vi "Alicat Comm Example.vi"() -> ()   [LabVIEW 2014, in "Alicat.lvlib"]
uses:
  Alicat.lvlib
  AlicatCommBank.lvclass
  MC/Alicat_MC.lvclass
  Alicat.lvclass
  Controls/Gas.ctl
  Controls/CtlSetup.ctl
  Data/MC/AlicatMCData.lvclass
panel:
  in  "SP1":dbl
  out "T 2":sgl
  out "P 2":sgl
  in  "SP":dbl[](array[numeric])
  out "P":sgl[](array[numeric])
  out "T":sgl[](array[numeric])
  in  "stop":bool
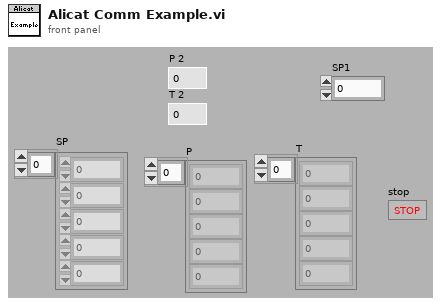
[diagram p1: front panel]
types:
  T1 = typedef "Alicat.lvlib/Alicat.lvclass/CtlSetup.ctl" = cluster{"Name":string, "Address":string, "fullScale":dbl, "Gas":T2}
  T2 = typedef "Alicat.lvlib/Alicat.lvclass/Gas.ctl" = enum16{"Air", "Ar", "CH4", "CO", "CO2", "C2H6", "H2", "He", "N2", "NO", "Ne", "O2", "C3H8", "n-C4H10", "C2H2", "C2H4", "i-C2H10", "Kr", "Xe"}
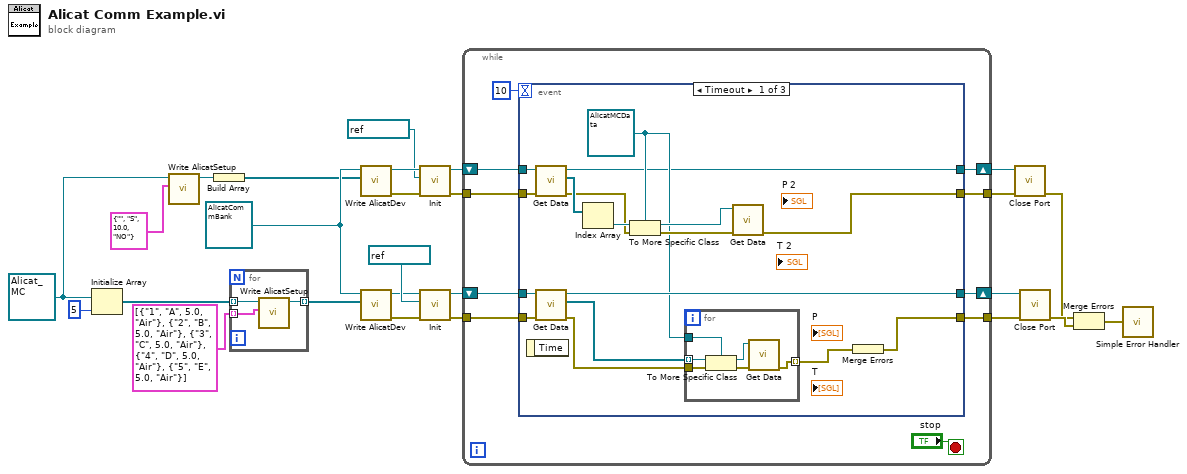
[diagram p0: block diagram]
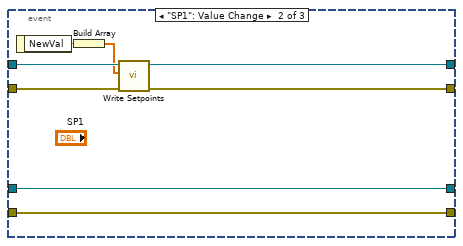
[diagram p2: hidden frame]
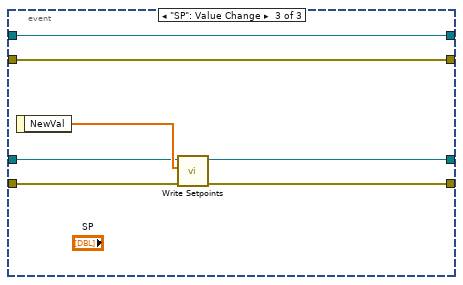
[diagram p3: hidden frame]
diagram:
  w15 = refnum<class "Alicat_MC.lvclass"> refnum ("Alicat_MC.lvclass")
  w12 = refnum<class "AlicatCommBank.lvclass"> refnum ("AlicatCommBank in")
  n1 = Initialize Array(w15, 5 ("dimension size")) -> (w18:refnum<class "Alicat_MC.lvclass">[])
  n2 = call "Write AlicatSetup.vi"("AlicatSetup"=T1 {"Name"="", "Address"="S", "fullScale"=10.0, "Gas"=enum."NO"}, "Alicat in"=w15) -> ("Alicat out"=w13:refnum<class "Alicat_MC.lvclass">)  [unwired: 8 in, 1 out]
  n3 = Build Array(w13) -> (w11:refnum<class "Alicat_MC.lvclass">[])
  n4 = for {
    tunnel: w18 -> [w29] mode=indexing
    tunnel: [w28] -> w17 mode=indexing
    tunnel: T1[] [{"Name"="1", "Address"="A", "fullScale"=5.0, "Gas"=enum."Air"}, {"Name"="2", "Address"="B", "fullScale"=5.0, "Gas"=enum."Air"}, {"Name"="3", "Address"="C", "fullScale"=5.0, "Gas"=enum."Air"}, {"Name"="4", "Address"="D", "fullScale"=5.0, "Gas"=enum."Air"}, {"Name"="5", "Address"="E", "fullScale"=5.0, "Gas"=enum."Air"}] -> [w27] mode=indexing
    n5 = call "Write AlicatSetup.vi"("AlicatSetup"=w27, "Alicat in"=w29) -> ("Alicat out"=w28:refnum<class "Alicat_MC.lvclass">)  [unwired: 8 in, 1 out]
  }
  n6 = call "Write AlicatDev.vi"("AlicatDev"=w11, "AlicatCommBank in"=w12) -> ("error out"=w7:errorcluster, "AlicatCommBank out"=w8:refnum<class "AlicatCommBank.lvclass">)  [unwired: 8 in]
  n7 = call "Write AlicatDev.vi"("AlicatDev"=w17, "AlicatCommBank in"=w12) -> ("error out"=w23:errorcluster, "AlicatCommBank out"=w25:refnum<class "AlicatCommBank.lvclass">)  [unwired: 8 in]
  n8 = call-dynamic "Init.vi"("error in"=w7, "Port"=refnum<visa-resource-name> "COM5", "AlicatCommBank in"=w8) -> ("error out"=w4:errorcluster, "AlicatCommBank out"=w5:refnum<class "AlicatCommBank.lvclass">)  [unwired: 7 in]
  n9 = call-dynamic "Init.vi"("error in"=w23, "Port"=refnum<visa-resource-name> "COM3", "AlicatCommBank in"=w25) -> ("error out"=w21:errorcluster, "AlicatCommBank out"=w22:refnum<class "AlicatCommBank.lvclass">)  [unwired: 7 in]
  n10 = while {
    tunnel: w21 -> [w38]
    tunnel: [w35] -> w19
    tunnel: w4 -> [w32]
    tunnel: [w30] -> w9
    shift-right: [w36] -> w20
    shift-left: w22 -> [w39]
    shift-right: [w31] -> w10
    shift-left: w5 -> [w33]
    stop <- "stop" stop-if-true
    n11 = event shown="[0] Timeout" {
      selector: _ -> [_ _ _]
      dyn-events: _ -> [_ _ _]
      timeout: 10 -> [_ _ _]
      tunnel: w39 -> [w56 w70 w76]
      tunnel: w38 -> [w55 w69 w75]
      tunnel: [w54 w70 w73] -> w36
      tunnel: [w40 w69 w74] -> w35
      tunnel: w33 -> [w52 w68 w72]
      tunnel: w32 -> [w51 w67 w71]
      tunnel: [w45 w65 w72] -> w31
      tunnel: [w43 w66 w71] -> w30
      event Timeout {
        w46 = refnum<class "AlicatMCData.lvclass"> refnum ("Alicat.lvlib:AlicatMCData.lvclass")
        n12 = event-data() -> ()  [unwired: 1 in, 1 out]
        n13 = call-dynamic "Get Data.vi"("error in"=w51, "AlicatCommBank in"=w52) -> ("error out"=w44:errorcluster, "DataOut"=w48:refnum<class "Data.lvclass">[], "AlicatCommBank out"=w45:refnum<class "AlicatCommBank.lvclass">)  [unwired: 7 in]
        n14 = call-dynamic "Get Data.vi"("error in"=w55, "AlicatCommBank in"=w56) -> ("error out"=w42:errorcluster, "DataOut"=w53:refnum<class "Data.lvclass">[], "AlicatCommBank out"=w54:refnum<class "AlicatCommBank.lvclass">)  [unwired: 7 in]
        n15 = Index Array(array=w48) -> (element=w47:refnum<class "Data.lvclass">)  [unwired: 1 in]
        n16 = To More Specific Class(target class=w46, reference=w47, error in=w44) -> (specific class reference=w50:refnum<class "AlicatMCData.lvclass">, error out=w49:errorcluster)
        n17 = for {
          tunnel: w53 -> [w61] mode=indexing
          tunnel: w46 -> [w60]
          tunnel: w42 -> [w58]
          tunnel: [w57] -> w41 mode=indexing
          n18 = To More Specific Class(target class=w60, reference=w61, error in=w58) -> (specific class reference=w59:refnum<class "AlicatMCData.lvclass">, error out=w62:errorcluster)
          n19 = call "Get Data.vi"("error in"=w62, "AlicatMData in"=w59) -> ("error out"=w57:errorcluster)  [unwired: 7 in, 2 out]
        }
        n20 = call "Get Data.vi"("error in"=w49, "AlicatMData in"=w50) -> ("error out"=w43:errorcluster)  [unwired: 7 in, 2 out]
        n21 = Merge Errors(w41) -> (w40:errorcluster)
      }
      event "SP1": Value Change {
        n22 = event-data() -> ("NewVal"=w64:dbl)  [unwired: 1 in]
        n23 = Build Array(w64) -> (w63:dbl[])
        n24 = call-dynamic "Write Setpoints.vi"("error in"=w67, "Setpoints"=w63, "AlicatCommBank in"=w68) -> ("error out"=w66:errorcluster, "AlicatCommBank out"=w65:refnum<class "AlicatCommBank.lvclass">)  [unwired: 7 in]
      }
      event "SP": Value Change {
        n25 = event-data() -> ("NewVal"=w77:dbl[])  [unwired: 1 in]
        n26 = call-dynamic "Write Setpoints.vi"("error in"=w75, "Setpoints"=w77, "AlicatCommBank in"=w76) -> ("error out"=w74:errorcluster, "AlicatCommBank out"=w73:refnum<class "AlicatCommBank.lvclass">)  [unwired: 7 in]
      }
    }
  }
  n27 = call-dynamic "Close Port.vi"("error in (no error)"=w9, "Serial IO in"=w10) -> ("error out"=w2:errorcluster)  [unwired: 8 in, 1 out]
  n28 = call-dynamic "Close Port.vi"("error in (no error)"=w19, "Serial IO in"=w20) -> ("error out"=w3:errorcluster)  [unwired: 8 in, 1 out]
  n29 = Merge Errors(w2, w3) -> (w1:errorcluster)
  n30 = call <vilib>:"Simple Error Handler.vi"("error in (no error)"=w1) -> ()  [unwired: 4 in, 5 out]
